vi "FileGlobalsCreate.vi"(3 "error in (no error)":errorcluster, 5 "Sequence Context":refnum<k7>) -> (0 "error out":errorcluster)   [LabVIEW 2015, in "ni-veristand-steps-runtime-lib.lvlib"]
uses:
  ni-veristand-steps-runtime-lib.lvlib
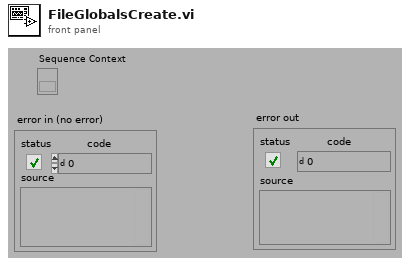
[diagram p1: front panel]
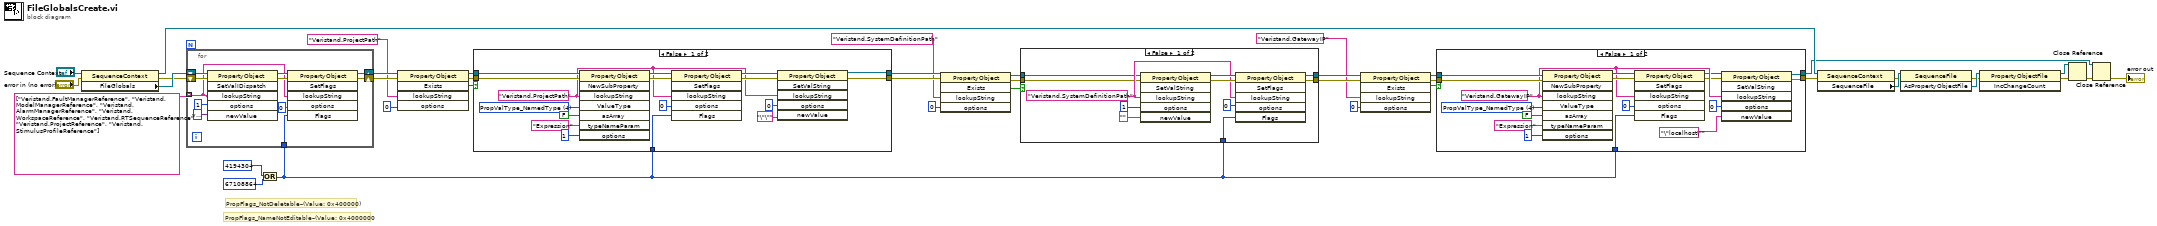
[diagram p0: block diagram]
diagram:
  # "PropFlags_NotDeletable–(Value: 0x400000)"
  # "PropFlags_NameNotEditable–(Value: 0x4000000"
  n1 = property class="SequenceContext"(reference="Sequence Context", error in="error in (no error)") -> (reference out=w38:refnum<k7>, error out=w29:errorcluster, "FileGlobals"=w40:refnum<k7>)
  n2 = Or(x=4194304 ("Flags"), y=67108864 ("Flags")) -> (x .or. y?=w22:i32)
  n3 = for {
    shift-right: [w45] -> w28
    shift-left: w40 -> [w51]
    tunnel: string[] ["Veristand.FaultManagerReference", "Veristand.ModelManagerReference", "Veristand.AlarmManagerReference", "Veristand.WorkspaceReference", "Veristand.RTSequenceReference", "Veristand.ProjectReference", "Veristand.StimulusProfileReference"] -> [w41] mode=indexing
    shift-right: [w44] -> w27
    shift-left: w29 -> [w48]
    tunnel: w22 -> [w43]
    n4 = invoke class="PropertyObject" method="SetValIDispatch"(reference=w51, error in=w48, "lookupString"=w41, "options"=1, "newValue"=variant) -> (reference out=w47:refnum<k7>, error out=w46:errorcluster)  [unwired: 1 in, 4 out]
    n5 = invoke class="PropertyObject" method="SetFlags"(reference=w47, error in=w46, "lookupString"=w41, "options"=0, "Flags"=w43) -> (reference out=w45:refnum<k7>, error out=w44:errorcluster)  [unwired: 1 in, 4 out]
  }
  n6 = invoke class="PropertyObject" method="Exists"(reference=w28, error in=w27, "lookupString"="Veristand.ProjectPath", "options"=0) -> (reference out=w4:refnum<k7>, error out=w5:errorcluster, "Exists"=w3:bool)  [unwired: 1 in, 2 out]
  n7 = case shown="False" w3 {
    tunnel: w4 -> [w68 w70]
    tunnel: w5 -> [w67 w69]
    tunnel: [w53 w69] -> w18
    tunnel: [w52 w70] -> w19
    tunnel: w22 -> [w60 _]
    frame False {
      w65 = 4 items=["PropValType_Container", "PropValType_String", "PropValType_Boolean", "PropValType_Number", "PropValType_NamedType", "PropValType_Reference", "PropValType_Array"] ("ValueType")
      w56 = "Veristand.ProjectPath"
      n8 = invoke class="PropertyObject" method="NewSubProperty"(reference=w68, error in=w67, "lookupString"=w56, "ValueType"=w65, "asArray"=FALSE, "typeNameParam"="Expression", "options"=1) -> (reference out=w62:refnum<k7>, error out=w61:errorcluster)  [unwired: 1 in, 6 out]
      n9 = invoke class="PropertyObject" method="SetFlags"(reference=w62, error in=w61, "lookupString"=w56, "options"=0, "Flags"=w60) -> (reference out=w58:refnum<k7>, error out=w57:errorcluster)  [unwired: 1 in, 4 out]
      n10 = invoke class="PropertyObject" method="SetValString"(reference=w58, error in=w57, "lookupString"=w56, "options"=0, "newValue"="\"\"") -> (reference out=w52:refnum<k7>, error out=w53:errorcluster)  [unwired: 1 in, 4 out]
    }
    frame True {
    }
  }
  n11 = invoke class="PropertyObject" method="Exists"(reference=w19, error in=w18, "lookupString"="Veristand.SystemDefinitionPath", "options"=0) -> (reference out=w9:refnum<k7>, error out=w8:errorcluster, "Exists"=w10:bool)  [unwired: 1 in, 2 out]
  n12 = case shown="False" w10 {
    tunnel: w22 -> [w75 _]
    tunnel: [w74 w82] -> w21
    tunnel: [w73 w83] -> w20
    tunnel: w9 -> [w72 w83]
    tunnel: w8 -> [w71 w82]
    frame False {
      w76 = "Veristand.SystemDefinitionPath"
      n13 = invoke class="PropertyObject" method="SetValString"(reference=w72, error in=w71, "lookupString"=w76, "options"=1, "newValue"="") -> (reference out=w78:refnum<k7>, error out=w77:errorcluster)  [unwired: 1 in, 4 out]
      n14 = invoke class="PropertyObject" method="SetFlags"(reference=w78, error in=w77, "lookupString"=w76, "options"=0, "Flags"=w75) -> (reference out=w73:refnum<k7>, error out=w74:errorcluster)  [unwired: 1 in, 4 out]
    }
    frame True {
    }
  }
  n15 = invoke class="PropertyObject" method="Exists"(reference=w20, error in=w21, "lookupString"="Veristand.GatewayIP", "options"=0) -> (reference out=w16:refnum<k7>, error out=w15:errorcluster, "Exists"=w17:bool)  [unwired: 1 in, 2 out]
  n16 = case shown="False" w17 {
    tunnel: w16 -> [w100 w102]
    tunnel: w15 -> [w99 w101]
    tunnel: [w85 w101] -> w23
    tunnel: [w84 w102] -> w24
    tunnel: w22 -> [w92 _]
    frame False {
      w97 = 4 items=["PropValType_Container", "PropValType_String", "PropValType_Boolean", "PropValType_Number", "PropValType_NamedType", "PropValType_Reference", "PropValType_Array"] ("ValueType")
      w88 = "Veristand.GatewayIP"
      n17 = invoke class="PropertyObject" method="NewSubProperty"(reference=w100, error in=w99, "lookupString"=w88, "ValueType"=w97, "asArray"=FALSE, "typeNameParam"="Expression", "options"=1) -> (reference out=w94:refnum<k7>, error out=w93:errorcluster)  [unwired: 1 in, 6 out]
      n18 = invoke class="PropertyObject" method="SetFlags"(reference=w94, error in=w93, "lookupString"=w88, "options"=0, "Flags"=w92) -> (reference out=w87:refnum<k7>, error out=w86:errorcluster)  [unwired: 1 in, 4 out]
      n19 = invoke class="PropertyObject" method="SetValString"(reference=w87, error in=w86, "lookupString"=w88, "options"=0, "newValue"="\"localhost\"") -> (reference out=w84:refnum<k7>, error out=w85:errorcluster)  [unwired: 1 in, 4 out]
    }
    frame True {
    }
  }
  n20 = property class="SequenceContext"(reference=w38, error in=w23) -> (error out=w36:errorcluster, "SequenceFile"=w37:refnum<k7>)  [unwired: 1 out]
  n21 = invoke class="SequenceFile" method="AsPropertyObjectFile"(reference=w37, error in=w36) -> (error out=w34:errorcluster, "AsPropertyObjectFile"=w35:refnum<k7>)  [unwired: 1 in, 1 out]
  n22 = invoke class="PropertyObjectFile" method="IncChangeCount"(reference=w35, error in=w34) -> (reference out=w32:refnum<k7>, error out=w33:errorcluster)  [unwired: 1 in, 1 out]
  n23 = Close Reference(reference=w32, error in (no error)=w33) -> (error out=w31:errorcluster)
  n24 = Close Reference(reference=w24, error in (no error)=w31) -> (error out=→"error out":errorcluster)
